vi "Get Firmware.vi"(0 "COM Port In":refnum<visa-resource-name>, 1 "error in":errorcluster) -> (2 "COM Port out":refnum<visa-resource-name>, 3 "Firmware":cluster{string, "read buffer":string}, 4 "OK":bool, 5 "error out":errorcluster)   [LabVIEW 2013]
doc: "The first action after opening the communication port should be to identify the laser/led we\nare connected to.\nThis will happen with the command “Get Firmware” (?GFw).\n\nThe answer will contain the model code, a device-ID and the firmware version of the device."
panel:
  out "Model Code":string
  out "Device ID":string
  out "Firmware":string
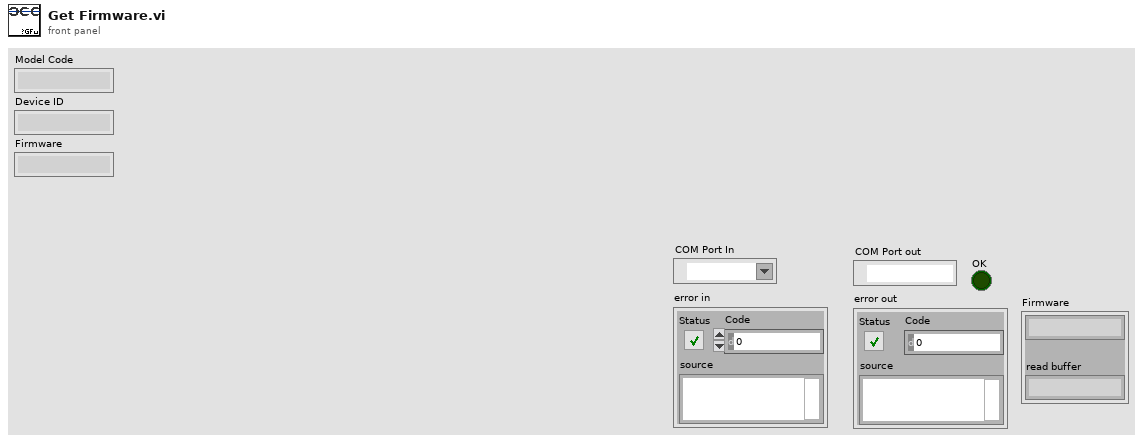
[diagram p1: front panel]
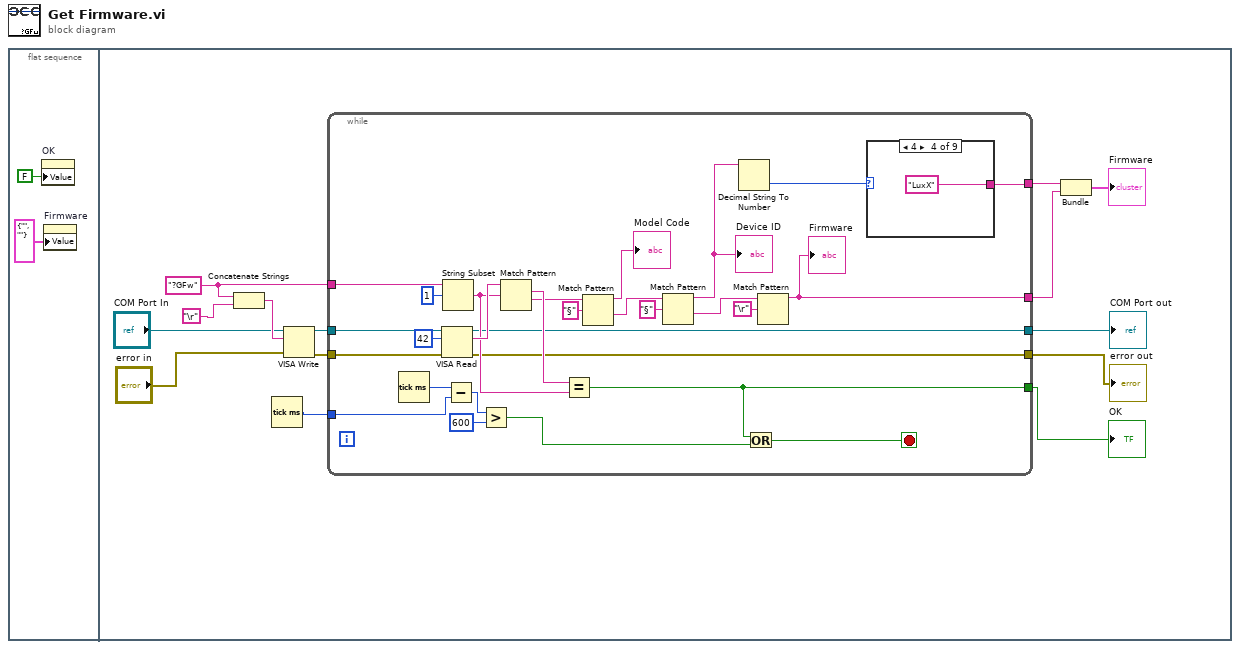
[diagram p0: block diagram]
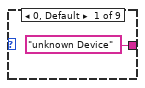
[diagram p2: hidden frame]
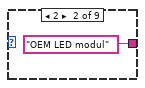
[diagram p3: hidden frame]
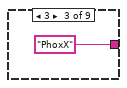
[diagram p4: hidden frame]
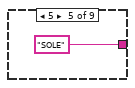
[diagram p5: hidden frame]
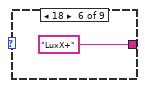
[diagram p6: hidden frame]
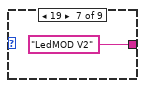
[diagram p7: hidden frame]
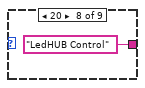
[diagram p8: hidden frame]
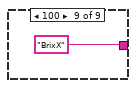
[diagram p9: hidden frame]
diagram:
  n1 = flat-sequence {
    frame #0 {
      n2 = property on="OK" class="Bool. (strikt)"("Value"=FALSE ("OK")) -> ()  [unwired: 2 in, 2 out]
      n3 = property on="Firmware" class="Cluster (strikt)"("Value"=cluster{string, "read buffer":string} {"", "read buffer"=""} ("Firmware")) -> ()  [unwired: 2 in, 2 out]
    }
    frame #1 {
      w5 = "?GFw" ("Schreibpuffer")
      n4 = Concatenate Strings(w5, "\r") -> (w11:string)
      n5 = Tick Count (ms)() -> (millisecond timer value=w3:u32)
      n6 = VISA Write(VISA resource name="COM Port In", write buffer=w11, error in (no error)="error in") -> (VISA resource name out=w6:refnum<visa-resource-name>, error out=w7:errorcluster)  [unwired: 1 out]
      n7 = while {
        tunnel: [w31] -> w16
        tunnel: [w30] -> w13
        tunnel: [w29] -> w12
        tunnel: [w27] -> w15
        tunnel: w7 -> [w26]
        tunnel: w6 -> [w23]
        tunnel: w5 -> [w25]
        tunnel: [w24] -> w4
        tunnel: w3 -> [w19]
        stop <- w28 stop-if-true
        n8 = Tick Count (ms)() -> (millisecond timer value=w20:u32)
        n9 = VISA Read(VISA resource name=w23, byte count=u32 42 ("Byte-Anzahl"), error in (no error)=w26) -> (VISA resource name out=w30:refnum<visa-resource-name>, read buffer=w40:string, error out=w29:errorcluster)  [unwired: 1 out]
        n10 = String Subset(string=w25, offset (0)=1 ("Offset (0)")) -> (substring=w34:string)  [unwired: 1 in]
        n11 = Subtract(x=w20, y=w19) -> (x-y=w21:u32)
        n12 = Greater?(x=w21, y=u32 600) -> (0:w18:bool)
        n13 = Match Pattern(string=w40, regular expression=w34) -> (match substring=w39:string, after substring=w38:string)  [unwired: 1 in, 2 out]
        n14 = Equal?(x=w39, y=w34) -> (x = y?=w24:bool)
        n15 = Match Pattern(string=w38, regular expression="§" ("Nach String/Zeichen suchen (-)")) -> (before substring=→"Model Code":string, after substring=w36:string)  [unwired: 1 in, 2 out]
        n16 = Match Pattern(string=w36, regular expression="§" ("Nach String/Zeichen suchen (-)")) -> (before substring=w33:string, after substring=w35:string)  [unwired: 1 in, 2 out]
        "Device ID" <- w33
        n17 = Decimal String To Number(string=w33) -> (number=w32:i32)  [unwired: 2 in, 1 out]
        n18 = Or(x=w24, y=w18) -> (x .or. y?=w28:bool)
        n19 = Match Pattern(string=w35, regular expression="\r") -> (before substring=w27:string)  [unwired: 1 in, 3 out]
        "Firmware" <- w27
        n20 = case shown="4" w32 {
          tunnel: ["unknown Device" "OEM LED modul" "PhoxX" "LuxX" "SOLE" "LuxX+" "LedMOD V2" "LedHUB Control" "BrixX"] -> w31
          frame 0, Default {
          }
          frame 2 {
          }
          frame 3 {
          }
          frame 4 {
          }
          frame 5 {
          }
          frame 18 {
          }
          frame 19 {
          }
          frame 20 {
          }
          frame 100 {
          }
        }
      }
      "OK" <- w4
      "COM Port out" <- w13
      "error out" <- w12
      n21 = Bundle(w16, "read buffer"=w15) -> (→"Firmware":cluster{string, "read buffer":string})  [unwired: 1 in]
    }
  }
